vi "Ex3Task5.vi"() -> ()   [LabVIEW 2014, in "Ex3Task1.lvrbt"]
uses:
  Ex3Task1.lvrbt
  <vilib>/NXT/Dual Mode Library/Sensors/EV3_Ultrasonic_CM.vi
panel:
  out "Error":bool
  in  "stop":bool
  out "Wall Proximity":string
  out "Current Distance":dbl
  in  "Min Distance":dbl
  in  "Max Distance":dbl
  out "Distance LED":bool
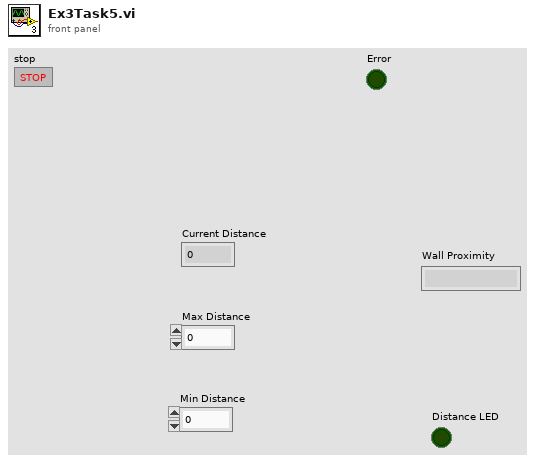
[diagram p1: front panel]
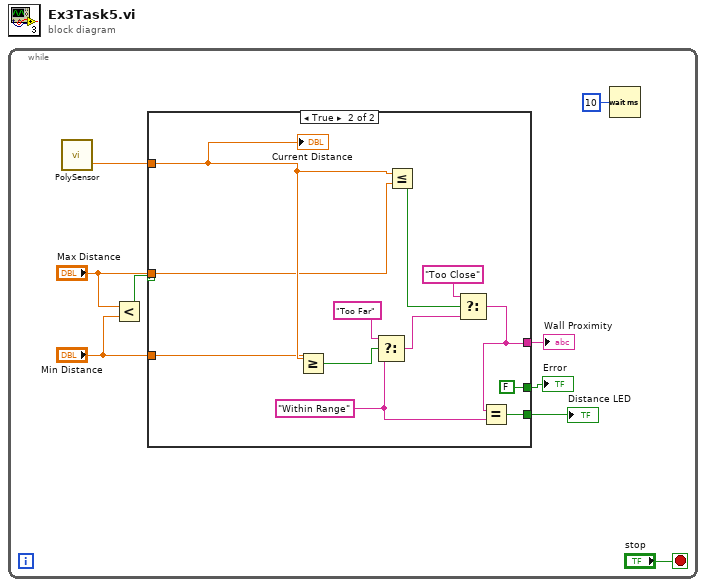
[diagram p0: block diagram]
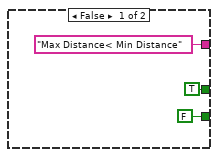
[diagram p2: hidden frame]
diagram:
  n1 = while {
    stop <- "stop" stop-if-true
    n2 = call-poly <vilib>:"PolySensor.vi"() -> ("Centimeters"=w7:sgl)  [unwired: 3 in, 1 out]
    n3 = Less?(x="Max Distance", y="Min Distance") -> (x < y?=w4:bool)
    n4 = case shown="True" w4 {
      tunnel: w7 -> [_ w24]
      tunnel: [FALSE w23] -> w6
      tunnel: ["Max Distance< Min Distance" w19] -> w5
      tunnel: "Max Distance" -> [_ w15]
      tunnel: "Min Distance" -> [_ w14]
      tunnel: [TRUE FALSE] -> w1
      frame False {
      }
      frame True {
        w16 = "Within Range"
        n5 = Greater Or Equal?(x=w24, y=w14) -> (x >= y?=w20:bool)
        n6 = Select(t="Too Far", s=w20, f=w16) -> (s? t:f=w22:string)
        n7 = Less Or Equal?(x=w24, y=w15) -> (x <= y?=w21:bool)
        n8 = Select(t="Too Close", s=w21, f=w22) -> (s? t:f=w19:string)
        n9 = Equal?(x=w19, y=w16) -> (x = y?=w23:bool)
        "Current Distance" <- w24
      }
    }
    "Distance LED" <- w6
    "Wall Proximity" <- w5
    "Error" <- w1
    n10 = Wait (ms)(milliseconds to wait=u32 10) -> ()  [unwired: 1 out]
  }
